vi "MOTOR TIMER.vi"() -> ()   [LabVIEW 2019]
uses:
  <vilib>/MakerHub/LINX/Public/Peripherals/Digital/Digital Write 1 Chan.vi
  <vilib>/MakerHub/LINX/Public/Peripherals/PWM/PWM Set Duty Cycle 1 Chan.vi
  <vilib>/MakerHub/LINX/Public/Peripherals/Digital/Digital Write N Chans.vi
  <vilib>/MakerHub/LINX/Private/Local IO/LinxDigitalWrite.vi
  <vilib>/MakerHub/LINX/Public/Utilities/Check Channel.vi
  <vilib>/MakerHub/LINX/Public/Utilities/Open Serial.vi
  <vilib>/MakerHub/LINX/Private/Utilties/Generate Error.vi
  <vilib>/MakerHub/LINX/Public/Peripherals/PWM/PWM Set Duty Cycle N Chans.vi
  <vilib>/MakerHub/LINX/LMH-LINX.lvlib
panel:
  in  "Stop Button":bool
  in  "DO Channel 5":u8
  in  "PWM Channel":u8
  in  "DO Channel":u8
  in  "Duty Cycle (0-1)":dbl
  in  "Serial Port":refnum<visa-resource-name>="N/A"
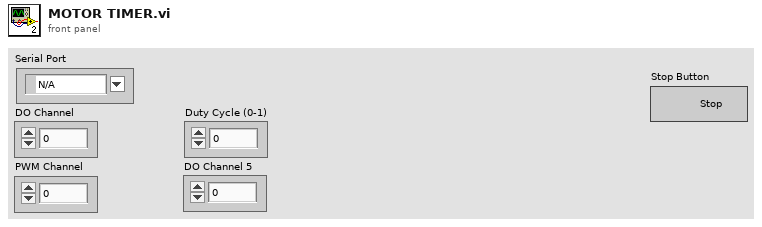
[diagram p1: front panel]
types:
  T1 = typedef "LMH-LINX.lvlib/LINX Ref.ctl" = cluster{"IO":T2, "Interface":T3, "LINX Device Config":T4}
  T2 = typedef "LMH-LINX.lvlib/Platform.ctl" = enum16{"Remote", "Local"}
  T3 = typedef "LMH-LINX.lvlib/Interface.ctl" = enum16{"Serial", "TCP"}
  T4 = typedef "LMH-LINX.lvlib/Device.lvlib/LINX Device Config.ctl" = cluster{"Interface":T3, "COM Port":refnum<visa-resource-name>, "TCP Configuration":T5, "Device Family":u8, "Device ID":u8, "Device Name":string, "TCP Ref":refnum<k5>, "Channels":T6}
  T5 = typedef "LMH-LINX.lvlib/Device.lvlib/TCP Config.ctl" = cluster{"IP Address":string, "Port":u16}
  T6 = typedef "LMH-LINX.lvlib/Channels.ctl" = cluster{"DI":u8[], "DO":u8[], "AI":u8[], "AO":u8[], "PWM":u8[], "QE":u8[], "UART":u8[], "I2C 2":u8[], "SPI":u8[], "CAN":u8[], "Servo":u8[], "AI Ref (V)":dbl, "AI Resolution (Bits)":u8, "AO Ref (V)":dbl, "AO Resolution (Bits)":u8}
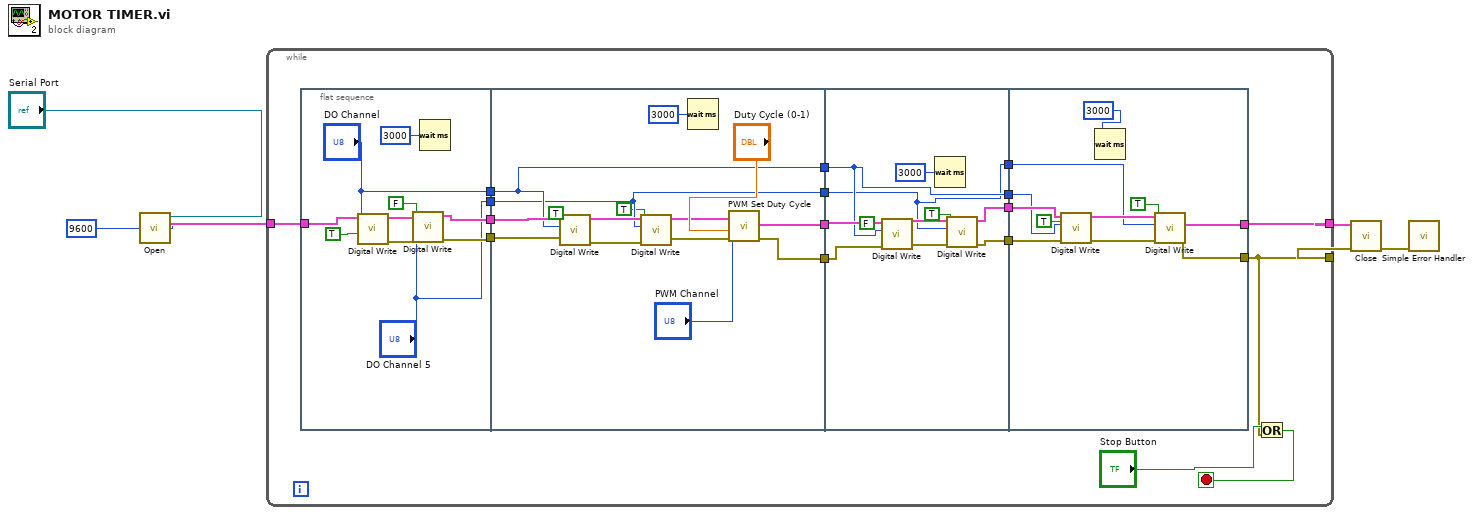
[diagram p0: block diagram]
diagram:
  n1 = call-poly <vilib>:"Open.vi"("Baud Rate Override"=u32 9600, "Serial Port"="Serial Port") -> ("LINX Resource"=w6:T1)  [unwired: 7 in, 2 out]
  n2 = while {
    tunnel: w6 -> [w23]
    tunnel: [w20] -> w3
    tunnel: [w7] -> w1
    stop <- w8 stop-if-true
    n3 = flat-sequence {
      tunnel: w23 -> [w33]
      tunnel: [w28] -> w22
      tunnel: [w27] -> w21
      tunnel: ["DO Channel 5"] -> w17
      tunnel: ["DO Channel"] -> w16
      tunnel: w22 -> [w47]
      tunnel: w21 -> [w48]
      tunnel: [w46] -> w19
      tunnel: [w45] -> w18
      tunnel: w17 -> [w35]
      tunnel: w16 -> [w36]
      tunnel: [w36] -> w15
      tunnel: [w35] -> w12
      tunnel: w19 -> [w58]
      tunnel: w18 -> [w59]
      tunnel: w15 -> [w50]
      tunnel: [w53] -> w14
      tunnel: [w52] -> w13
      tunnel: w12 -> [w49]
      tunnel: [w50] -> w11
      tunnel: [w49] -> w10
      tunnel: [w64] -> w20
      tunnel: [w63] -> w7
      tunnel: w14 -> [w68]
      tunnel: w13 -> [w67]
      tunnel: w11 -> [w62]
      tunnel: w10 -> [w61]
      frame #0 {
        n4 = call-poly <vilib>:"Digital Write.vi"("Output Value"=TRUE, "DO Channel"="DO Channel", "LINX Resource"=w33) -> ("Error Out"=w30:errorcluster, "LINX Resource"=w29:T1)  [unwired: 7 in]
        n5 = call-poly <vilib>:"Digital Write.vi"("Error In"=w30, "Output Value"=FALSE, "DO Channel"="DO Channel 5", "LINX Resource"=w29) -> ("Error Out"=w27:errorcluster, "LINX Resource"=w28:T1)  [unwired: 6 in]
        n6 = Wait (ms)(milliseconds to wait=u32 3000) -> ()  [unwired: 1 out]
      }
      frame #1 {
        n7 = call-poly <vilib>:"Digital Write.vi"("Error In"=w48, "Output Value"=TRUE, "DO Channel"=w36, "LINX Resource"=w47) -> ("Error Out"=w40:errorcluster, "LINX Resource"=w39:T1)  [unwired: 6 in]
        n8 = call-poly <vilib>:"Digital Write.vi"("Error In"=w40, "Output Value"=TRUE, "DO Channel"=w35, "LINX Resource"=w39) -> ("Error Out"=w37:errorcluster, "LINX Resource"=w38:T1)  [unwired: 6 in]
        n9 = Wait (ms)(milliseconds to wait=u32 3000) -> ()  [unwired: 1 out]
        n10 = call-poly <vilib>:"PWM Set Duty Cycle.vi"("Error In"=w37, "Duty Cycle (0-1)"="Duty Cycle (0-1)", "PWM Channel"="PWM Channel", "LINX Resource"=w38) -> ("Error Out"=w46:errorcluster, "LINX Resource"=w45:T1)  [unwired: 6 in]
      }
      frame #2 {
        n11 = call-poly <vilib>:"Digital Write.vi"("Error In"=w58, "Output Value"=FALSE, "DO Channel"=w50, "LINX Resource"=w59) -> ("Error Out"=w54:errorcluster, "LINX Resource"=w55:T1)  [unwired: 6 in]
        n12 = Wait (ms)(milliseconds to wait=u32 3000) -> ()  [unwired: 1 out]
        n13 = call-poly <vilib>:"Digital Write.vi"("Error In"=w54, "Output Value"=TRUE, "DO Channel"=w49, "LINX Resource"=w55) -> ("Error Out"=w52:errorcluster, "LINX Resource"=w53:T1)  [unwired: 6 in]
      }
      frame #3 {
        n14 = call-poly <vilib>:"Digital Write.vi"("Error In"=w67, "Output Value"=TRUE, "DO Channel"=w62, "LINX Resource"=w68) -> ("Error Out"=w65:errorcluster, "LINX Resource"=w66:T1)  [unwired: 6 in]
        n15 = Wait (ms)(milliseconds to wait=u32 3000) -> ()  [unwired: 1 out]
        n16 = call-poly <vilib>:"Digital Write.vi"("Error In"=w65, "Output Value"=TRUE, "DO Channel"=w61, "LINX Resource"=w66) -> ("Error Out"=w63:errorcluster, "LINX Resource"=w64:T1)  [unwired: 6 in]
      }
    }
    n17 = Or(x="Stop Button", y=w7) -> (x .or. y?=w8:bool)
  }
  n18 = call <vilib>:"Close.vi"("Error In"=w1, "LINX Resource"=w3) -> ("Error Out"=w2:errorcluster)  [unwired: 9 in]
  n19 = call <vilib>:"Simple Error Handler.vi"("error in (no error)"=w2) -> ()  [unwired: 4 in, 5 out]
